vi "Condition Valid Control In Terminal.vi"(6 "Control":refnum<vi>, 9 "Terminal":i32, 10 "Terminals":T1) -> (2 "Valid":bool)   [LabVIEW 2025, in "_Rescript.lvlib"]
uses:
  Msg/Msg/Msg.lvclass/Msg.ctl
  _Rescript.lvlib
  Terminals.ctl
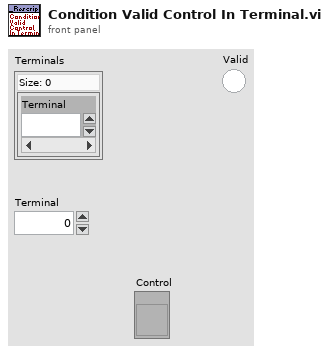
[diagram p1: front panel]
types:
  T1 = typedef "_Rescript.lvlib/Terminals.ctl" = set{i32}
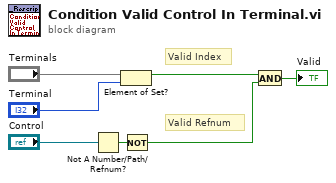
[diagram p0: block diagram]
diagram:
  # "Valid Refnum"
  # "Valid Index"
  n1 = Not A Number/Path/Refnum?(number/path/refnum="Control") -> (NaN/Path/Refnum?=w7:bool)
  n2 = Element of Set?(10:"Terminal", 11:"Terminals") -> (3:w1:bool)
  n3 = Not(x=w7) -> (.not. x?=w6:bool)
  n4 = And(x=w1, y=w6) -> (x .and. y?=→"Valid":bool)
